vi "Save_Data_To_File.vi"(6 "Save Header?":bool, 8 "error in (no error)":errorcluster, 10 "Filepath Input":path, 11 "Data Array in":string[][](array[string])) -> (0 "error out":errorcluster, 2 "Filepath Output":path, 4 "Save Header Out?":bool)   [LabVIEW 2023]
uses:
  <vilib>/Utility/file.llb/Write Delimited Spreadsheet (string).vi
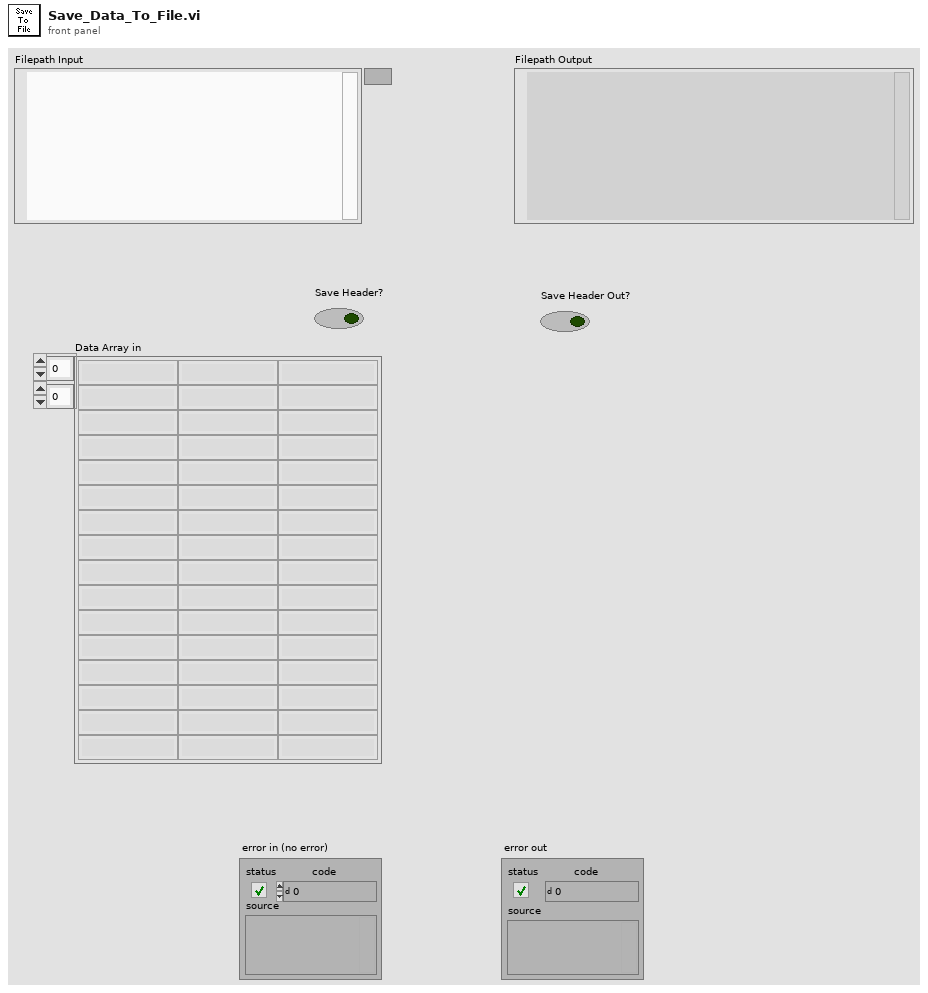
[diagram p1: front panel]
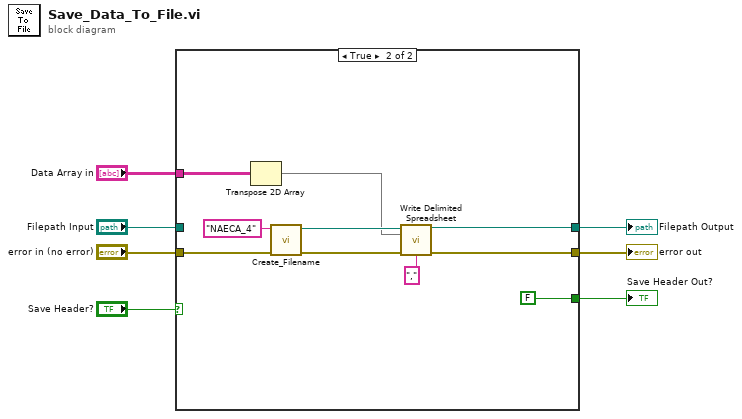
[diagram p0: block diagram]
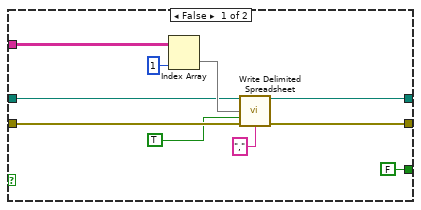
[diagram p2: hidden frame]
diagram:
  n1 = case shown="True" "Save Header?" {
    tunnel: [FALSE FALSE] -> w6
    tunnel: "Data Array in" -> [w13 w19]
    tunnel: "error in (no error)" -> [w15 w24]
    tunnel: [w14 w25] -> w3
    tunnel: [w9 w20] -> w2
    tunnel: "Filepath Input" -> [w10 _]
    frame False {
      n2 = Index Array(array=w13, index (col)=1 ("disabled index (col)")) -> (element=w12:string[])  [unwired: 1 in]
      n3 = call-poly <vilib>:"Write Delimited Spreadsheet.vi"("file path (dialog if empty)"=w10, "1D data"=w12, "append to file? (new file:F)"=TRUE, "error in (no error)"=w15, "delimiter (\\t)"="," ("delimiter (\\t)")) -> ("new file path (Not A Path if cancelled)"=w9:path, "error out"=w14:errorcluster)  [unwired: 9 in]
    }
    frame True {
      n4 = Transpose 2D Array(2D array=w19) -> (transposed array=w18:string[][])
      n5 = call "Create_Filename.vi"("error in (no error)"=w24, "Test string input"="NAECA_4") -> ("error out"=w23:errorcluster, "path for csv file"=w22:path)  [unwired: 8 in]
      n6 = call-poly <vilib>:"Write Delimited Spreadsheet.vi"("file path (dialog if empty)"=w22, "2D data"=w18, "error in (no error)"=w23, "delimiter (\\t)"="," ("delimiter (\\t)")) -> ("new file path (Not A Path if cancelled)"=w20:path, "error out"=w25:errorcluster)  [unwired: 10 in]
    }
  }
  "error out" <- w3
  "Save Header Out?" <- w6
  "Filepath Output" <- w2
